vi "Display.vi"(8 "error in":errorcluster, 11 "Plain - Two Button in":refnum<class "Plain - Two Button.lvclass">) -> (0 "error out":errorcluster, 3 "Plain - Two Button out":refnum<class "Plain - Two Button.lvclass">)   [LabVIEW 2021, in "Pop-Up.lvlib" / "Plain - Two Button.lvclass"]
doc: "This is the override method required for each child of the pop up class. It is the pop up that will display to the user.\n\nTo extend this function, create a child class of the pop up class. Then create an override method for this VI. <b>Display.vi</b> is a protected function, therefore it cannot be called in a main application. This VI must be called by a caller function. See one of the standard pop-ups for a setup example.\n\n<b>Code Developed By:</b> +\nDaniel Coons +\nhttps://github.com/danielcoons/tsc-pop-up"
uses:
  Plain - Two Button.lvclass
  C:/Development/Open Source/tsc-pop-up/Popup/Popup.lvclass
  C:/Development/Open Source/tsc-pop-up/Plain/Plain Parent.lvclass
  Popup/Popup.lvclass/Popup.ctl
  Plain Parent.lvclass/Plain Parent.ctl
  Popup/Data Member Access/Read Theme.vi
  Read Dialog Title.vi
  Read Action 1 Text.vi
  Read Action 2 Text.vi
  Theme/Theme.lvclass
  Plain - Two Button.lvclass/Plain - Two Button.ctl
  Popup/Popup.lvclass
  user32.dll
panel:
  in  "action 2":bool
  out "dialog title":string
  out "message":string
  in  "action 1":bool
  # "This VI displays the popup"
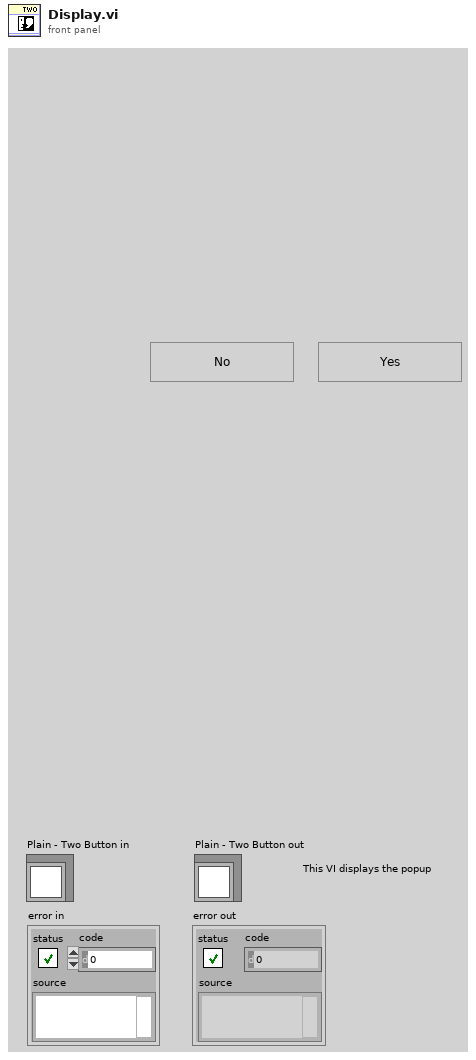
[diagram p1: front panel]
types:
  T1 = typedef "LVRectTypeDef.ctl" = cluster{"Left":i16, "Top":i16, "Right":i16, "Bottom":i16}
  T2 = typedef "LVPointTypeDef.ctl" = cluster{"Horizontal":i16, "Vertical":i16}
  T3 = typedef "LVPoint32TypeDef.ctl" = cluster{"Horizontal":i32, "Vertical":i32}
  T4 = typedef "LVPositionTypeDef.ctl" = cluster{"Left":i32, "Top":i32}
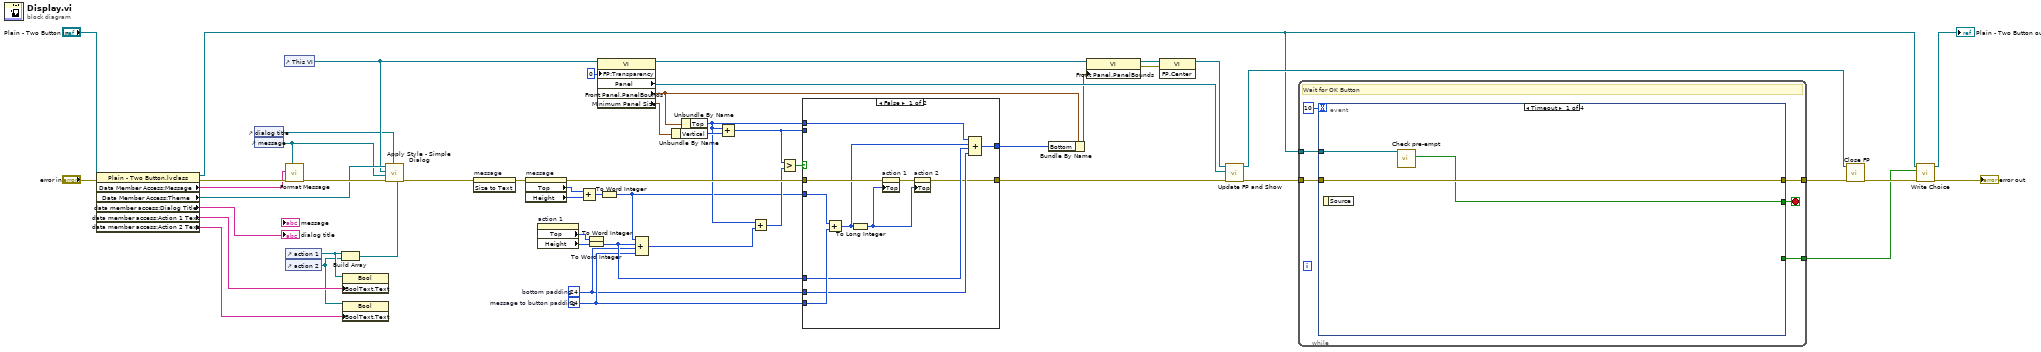
[diagram p0: block diagram]
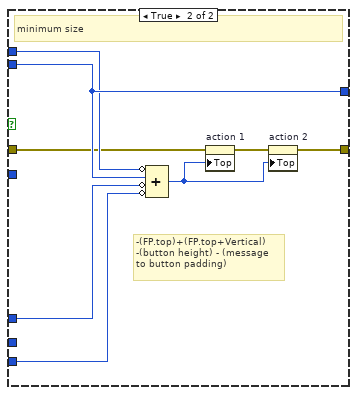
[diagram p2: hidden frame]
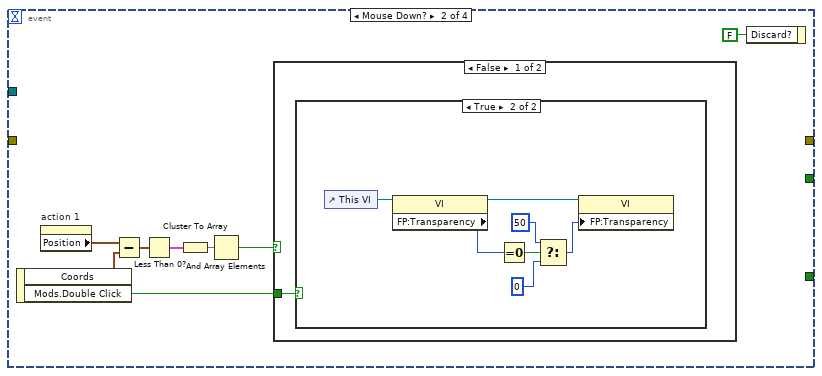
[diagram p3: hidden frame]
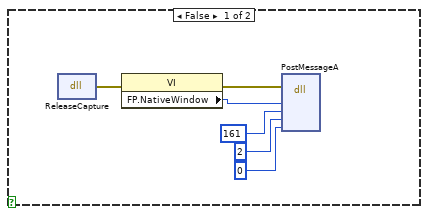
[diagram p4: hidden frame]
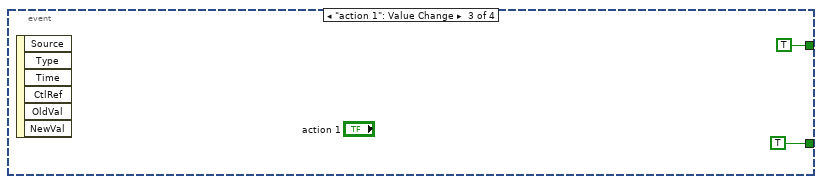
[diagram p6: hidden frame]
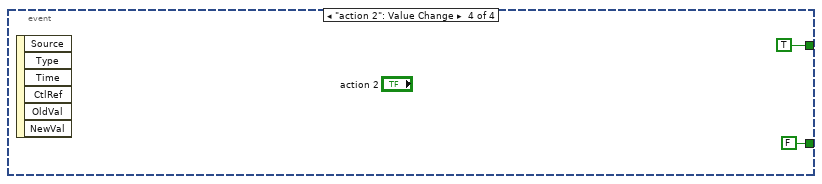
[diagram p7: hidden frame]
diagram:
  w27 = i16 24  # message to button padding
  w25 = i16 24  # bottom padding
  n1 = property class="Plain - Two Button.lvclass"(reference="Plain - Two Button in", error in="error in") -> (reference out=w7:refnum<class "Plain - Two Button.lvclass">, error out=w48:errorcluster, "Data Member Access:Message"=w46:string, "Data Member Access:Theme"=w19:refnum<class "Theme.lvclass">, "data member access:Dialog Title"=→"dialog title":string, "data member access:Action 1 Text"=w14:string, "data member access:Action 2 Text"=w9:string)
  n2 = control-ref of="dialog title"() -> (w4:refnum<vi>)
  n3 = control-ref of="message"() -> (w3:refnum<vi>)
  n4 = control-ref of="This VI"() -> (w18:refnum<vi>)
  n5 = call "Format Message.vi"("formatted string"=w3, "error in"=w48, "String Input"=w46) -> ("error out"=w21:errorcluster)  [unwired: 7 in, 1 out]
  n6 = control-ref of="action 1"() -> (w15:refnum<vi>)
  n7 = control-ref of="action 2"() -> (w10:refnum<vi>)
  n8 = Build Array(w15, w10) -> (w17:refnum<vi>[])
  n9 = property class="Bool"(reference=w15, "BoolText.Text"=w14) -> ()  [unwired: 1 in, 2 out]
  n10 = property class="Bool"(reference=w10, "BoolText.Text"=w9) -> ()  [unwired: 1 in, 2 out]
  n11 = call "Apply Style - Simple Dialog.vi"("button refs"=w17, "title ref"=w4, "error in"=w21, "message ref"=w3, "pop up ref"=w18, "Theme in"=w19) -> ("error out"=w20:errorcluster)  [unwired: 4 in, 1 out]
  n12 = invoke on="message" class="Str" method="Size to Text"(error in=w20) -> (error out=w47:errorcluster)  [unwired: 2 in, 2 out]
  n13 = property on="message" class="Str"(error in=w47) -> (error out=w30:errorcluster, "Top"=w41:i32, "Height"=w40:u32)  [unwired: 1 in, 1 out]
  n14 = property on="action 1" class="Bool"() -> ("Top"=w43:i32, "Height"=w42:u32)  [unwired: 2 in, 2 out]
  n15 = Add(x=w41, y=w40) -> (x+y=w39:u32)
  n16 = To Word Integer(number=w43) -> ()  [unwired: 1 out]
  n17 = To Word Integer(number=w42) -> (16bit integer=w28:i16)
  n18 = property class="VI"(reference=w18, "FP:Transparency"=u8 0 ("Front Panel Window:Transparency")) -> (reference out=w45:refnum<vi>, "Panel"=w44:refnum<vi>, "Front Panel.PanelBounds"=w35:T1, "Minimum Panel Size"=w38:T2)  [unwired: 1 in, 1 out]
  n19 = To Word Integer(number=w39) -> (16bit integer=w2:i16)
  n20 = Compound Arithmetic op=ADD(w2, w28, w25, w27) -> (w1:i16)
  n21 = Unbundle By Name(w38) -> ("Vertical"=w37:i16)
  n22 = Unbundle By Name(w35) -> ("Top"=w22:i16)
  n23 = Add(x=w22, y=w37) -> (x+y=w23:i16)
  n24 = Add(x=w22, y=w1) -> (x+y=w24:i16)
  n25 = Greater?(x=w23, y=w24) -> (0:w31:bool)
  n26 = case shown="False" w31 {
    tunnel: [w62 w71] -> w26
    tunnel: w23 -> [_ w71]
    tunnel: w2 -> [w63 _]
    tunnel: w22 -> [w56 w70]
    tunnel: w30 -> [w61 w69]
    tunnel: [w54 w65] -> w29
    tunnel: w28 -> [w58 w68]
    tunnel: w27 -> [w60 w67]
    tunnel: w25 -> [w59 _]
    frame False {
      n27 = Add(x=w63, y=w60) -> (x+y=w57:i16)
      n28 = To Long Integer(number=w57) -> (32bit integer=w53:i32)
      n29 = property on="action 1" class="Bool"(error in=w61, "Top"=w53) -> (error out=w55:errorcluster)  [unwired: 1 in, 1 out]
      n30 = property on="action 2" class="Bool"(error in=w55, "Top"=w53) -> (error out=w54:errorcluster)  [unwired: 1 in, 1 out]
      n31 = Compound Arithmetic op=ADD(w56, w57, w58, w59) -> (w62:i16)
    }
    frame True {
      # "-(FP.top)+(FP.top+Vertical)\n-(button height) - (message\nto button padding)"
      # "minimum size"
      n32 = Compound Arithmetic op=ADD(invert w70, w71, invert w68, invert w67) -> (w64:i16)
      n33 = property on="action 1" class="Bool"(error in=w69, "Top"=w64) -> (error out=w66:errorcluster)  [unwired: 1 in, 1 out]
      n34 = property on="action 2" class="Bool"(error in=w66, "Top"=w64) -> (error out=w65:errorcluster)  [unwired: 1 in, 1 out]
    }
  }
  n35 = Bundle By Name(cluster=w35, "Bottom"=w26) -> (w32:T1)
  n36 = property class="VI"(reference=w45, "Front Panel.PanelBounds"=w32) -> (reference out=w36:refnum<vi>, error out=w33:errorcluster)  [unwired: 1 in]
  n37 = invoke class="VI" method="FP.Center"(reference=w36, error in=w33) -> (reference out=w34:refnum<vi>)  [unwired: 1 in, 2 out]
  n38 = call "Update FP and Show.vi"("error in (no error)"=w29, "Panel Ref"=w44, "VI in"=w34) -> ("error out"=w51:errorcluster, "VI out"=w50:refnum<vi>)  [unwired: 7 in]
  n39 = while {
    tunnel: [w75] -> w52
    tunnel: w51 -> [w76]
    tunnel: w7 -> [w73]
    tunnel: [w72] -> w6
    stop <- w77 stop-if-true
    # "Wait for OK Button"
    n40 = event shown="[0] Timeout" {
      selector: _ -> [_ _ _ _]
      dyn-events: _ -> [_ _ _ _]
      timeout: 10 -> [_ _ _ _]
      tunnel: [w78 _ TRUE ("Pre-empted?") TRUE ("Pre-empted?")] -> w77
      tunnel: w76 -> [w80 _ _ _]
      tunnel: [w80 _ _ _] -> w75
      tunnel: w73 -> [w79 _ _ _]
      tunnel: [_ _ TRUE FALSE] -> w72
      event Timeout {
        n41 = event-data() -> ()  [unwired: 1 in, 1 out]
        n42 = call "Check pre-empt.vi"("_Popup in"=w79) -> ("Pre-empted?"=w78:bool)  [unwired: 8 in, 2 out]
      }
      event Mouse Down? {
        n43 = event-data() -> ("Coords"=w82:T3, "Mods.Double Click"=w84:bool)  [unwired: 1 in]
        n44 = property on="action 1" class="Bool"() -> ("Position"=w83:T4)  [unwired: 2 in, 2 out]
        n45 = Subtract(x=w83, y=w82) -> (x-y=w85:T4)
        n46 = Less Than 0?(x=w85) -> (x < 0?=w86:cluster{"Left":bool, "Top":bool})
        n47 = Cluster To Array(cluster=w86) -> (array=w87:bool[])
        n48 = And Array Elements(Boolean array=w87) -> (logical AND=w88:bool)
        n49 = case shown="False" w88 {
          tunnel: w84 -> [w89 _]
          frame False {
            n50 = case shown="True" w89 {
              frame False {
                n51 = dll-call lib="user32.dll" fn="ReleaseCapture"() -> (error out=w93:errorcluster)  [unwired: 4 in, 1 out]
                n52 = property class="VI"(error in=w93) -> (error out=w94:errorcluster, "FP.NativeWindow"=w95:u64)  [unwired: 1 in, 1 out]
                n53 = dll-call lib="user32.dll" fn="PostMessageA"(error in=w94, "hWnd"=w95, "Msg"=161, "wParam"=2, "lParam"=0) -> ()  [unwired: 7 in, 2 out]
              }
              frame True {
                n54 = control-ref of="This VI"() -> (w102:refnum<vi>)
                n55 = property class="VI"(reference=w102) -> (reference out=w100:refnum<vi>, "FP:Transparency"=w101:u8)  [unwired: 1 in, 1 out]
                n56 = Equal To 0?(x=w101) -> (x = 0?=w99:bool)
                n57 = Select(t=u8 50, s=w99, f=u8 0) -> (s? t:f=w98:u8)
                n58 = property class="VI"(reference=w100, "FP:Transparency"=w98) -> ()  [unwired: 1 in, 2 out]
              }
            }
          }
          frame True {
          }
        }
        n59 = event-data("Discard?"=FALSE) -> ()  [unwired: 1 in, 1 out]
      }
      event "action 1": Value Change {
        n60 = event-data() -> ()  [unwired: 1 in, 6 out]
      }
      event "action 2": Value Change {
        n61 = event-data() -> ()  [unwired: 1 in, 6 out]
      }
    }
  }
  n62 = call "Close FP.vi"("error in (no error)"=w52, "VI in"=w50) -> ("error out"=w13:errorcluster)  [unwired: 9 in]
  n63 = call-dynamic "Write Choice.vi"("error in (no error)"=w13, "Choice"=w6, "_Popup in"=w7) -> ("error out"=→"error out":errorcluster, "_Popup out"=→"Plain - Two Button out":refnum<class "Plain - Two Button.lvclass">)  [unwired: 7 in]
